vi "AddData.vi"(0 "SettingsFileList in":refnum<class "SettingsFileList.lvclass">, 1 "ProjectName":string, 2 "FileName":string, 3 "MD5 (optional)":string, 4 "BinaryData":string, 5 "error in (no error)":errorcluster) -> (14 "SettingsFileList out":refnum<class "SettingsFileList.lvclass">, 15 "MD5 is same":bool, 19 "error out":errorcluster)   [LabVIEW 2018, in "SettingsFileList.lvclass"]
uses:
  SettingsFileList.lvclass
  SettingsFile.lvclass
  SettingsFileList.lvclass/SettingsFileList.ctl
  SettingsFile.lvclass/SettingsFile.ctl
panel:
  out "SettingsFile out":refnum<class "SettingsFile.lvclass">
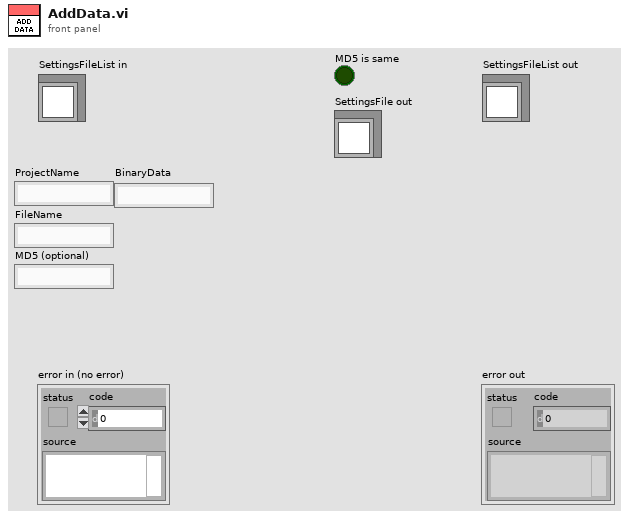
[diagram p1: front panel]
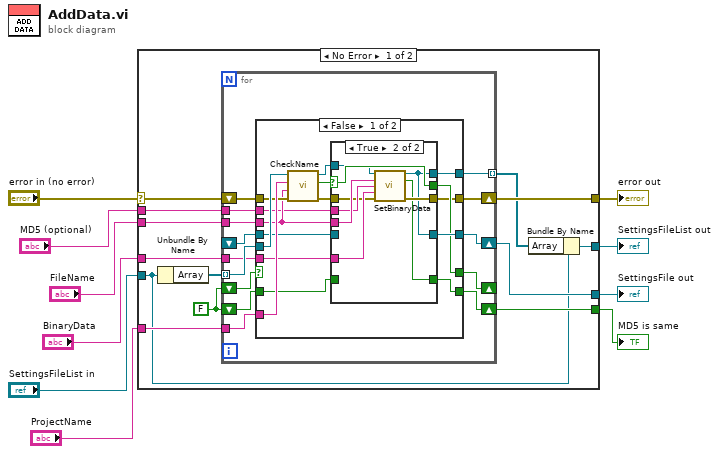
[diagram p0: block diagram]
diagram:
  n1 = case shown="No Error" "error in (no error)" {
    selector: "error in (no error)" -> [w19 w74]
    tunnel: [w18 w74] -> w9
    tunnel: [w20 _] -> w4
    tunnel: "SettingsFileList in" -> [w12 w73]
    tunnel: "ProjectName" -> [w22 _]
    tunnel: "FileName" -> [w21 _]
    tunnel: "MD5 (optional)" -> [w17 _]
    tunnel: "BinaryData" -> [w16 _]
    tunnel: [w15 _] -> w2
    tunnel: [w11 w73] -> w1
    frame No Error {
      w14 = FALSE
      n2 = Unbundle By Name(w12) -> ("Array"=w23:refnum<class "SettingsFile.lvclass">[])
      n3 = for {
        tunnel: w23 -> [w37] mode=indexing
        shift-right: [w31] -> _
        shift-left: w14 -> [w33]
        tunnel: w22 -> [w35]
        tunnel: w21 -> [w36]
        shift-right: [w34] -> w20
        shift-left: _ -> [w32]
        shift-right: [w29] -> w18
        shift-left: w19 -> [w30]
        tunnel: w17 -> [w28]
        tunnel: w16 -> [w27]
        shift-right: [w26] -> w15
        shift-left: w14 -> [w25]
        tunnel: [w24] -> w13 mode=indexing
        n4 = case shown="False" w33 {
          selector: w33 -> [_ w71]
          tunnel: w37 -> [w53 w68]
          tunnel: w36 -> [w43 _]
          tunnel: w35 -> [w52 _]
          tunnel: [w50 w72] -> w34
          tunnel: w32 -> [w48 w72]
          tunnel: [w47 w71] -> w31
          tunnel: w30 -> [w45 w70]
          tunnel: [w44 w70] -> w29
          tunnel: w28 -> [w42 _]
          tunnel: w27 -> [w41 _]
          tunnel: [w40 w69] -> w26
          tunnel: w25 -> [w39 w69]
          tunnel: [w38 w68] -> w24
          frame False {
            n5 = call "CheckName.vi"("error in (no error)"=w45, "FileName"=w43, "ProjectName"=w52, "SettingsFile in"=w53) -> ("error out"=w46:errorcluster, "Boolean"=w49:bool, "SettingsFile out"=w51:refnum<class "SettingsFile.lvclass">)  [unwired: 5 in]
            n6 = case shown="True" w49 {
              selector: w49 -> [w57 w67]
              tunnel: [w58 w59] -> w50
              tunnel: w51 -> [w54 w66]
              tunnel: w48 -> [w58 _]
              tunnel: [w57 w67] -> w47
              tunnel: w46 -> [w56 w62]
              tunnel: [w56 w61] -> w44
              tunnel: w43 -> [_ w65]
              tunnel: w42 -> [_ w64]
              tunnel: w41 -> [_ w63]
              tunnel: [w55 w60] -> w40
              tunnel: w39 -> [w55 _]
              tunnel: [w54 w59] -> w38
              frame False {
              }
              frame True {
                n7 = call "SetBinaryData.vi"("SettingsFile in"=w66, "FileName"=w65, "MD5"=w64, "BinaryData"=w63, "error in (no error)"=w62) -> ("SettingsFile out"=w59:refnum<class "SettingsFile.lvclass">, "MD5 is same"=w60:bool, "error out"=w61:errorcluster)  [unwired: 8 in]
              }
            }
          }
          frame True {
          }
        }
      }
      n8 = Bundle By Name(cluster=w12, "Array"=w13) -> (w11:refnum<class "SettingsFileList.lvclass">)
    }
    frame Error {
    }
  }
  "error out" <- w9
  "SettingsFileList out" <- w1
  "SettingsFile out" <- w4
  "MD5 is same" <- w2
